vi "SGUI Search Control Ref.vi"(6 "error in":errorcluster, 8 "control label (empty)":string, 9 "generate error if not found? (True)":bool=TRUE) -> (7 "error out":errorcluster, 10 "found?":bool, 11 "control ref out":refnum<vi>)   [LabVIEW 2013, in "varilib.lvlib"]
doc: "This VI searches control reference by its label in the previously regitered list (see 'SGUI Register Controls').\nIf multiple controls with the same name are found the priority has the last registered.\n\nError input is ignored however by default it will generate error if control is not found."
uses:
  varilib.lvlib
  SGUI Global Var.vi
  <vilib>/Utility/error.llb/Error Cluster From Error Code.vi
  <vilib>/ErrorRing/Error Ring.xnode
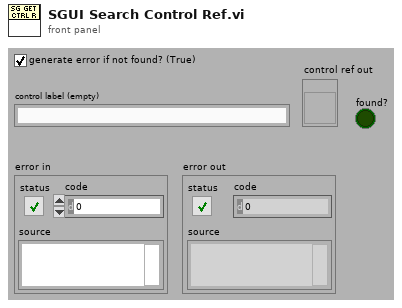
[diagram p1: front panel]
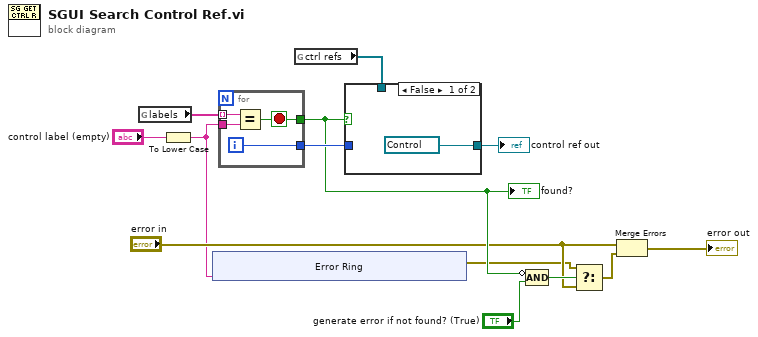
[diagram p0: block diagram]
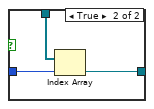
[diagram p2: hidden frame]
diagram:
  n1 = global read "SGUI Global Var.vi" "labels"() -> (w13:string[])
  n2 = To Lower Case(string="control label (empty)") -> (all lower case string=w1:string)
  n3 = xnode "Error Ring"("parameter 0"=w1) -> ("error out"=w2:errorcluster)
  n4 = for {
    tunnel: w13 -> [w17] mode=indexing
    tunnel: w1 -> [w16]
    tunnel: [w15] -> w11
    tunnel: [w14] -> w5
    i -> [w15]
    stop <- w14 stop-if-true
    n5 = Equal?(x=w17, y=w16) -> (x = y?=w14:bool)
  }
  "found?" <- w5
  n6 = global read "SGUI Global Var.vi" "ctrl refs"() -> (w12:refnum<vi>[])
  n7 = case shown="False" w5 {
    tunnel: w12 -> [_ w21]
    tunnel: w11 -> [_ w20]
    tunnel: [refnum<vi> refnum ("ctrl ref out") w19] -> w10
    frame False {
    }
    frame True {
      n8 = Index Array(array=w21, index=w20) -> (element=w19:refnum<vi>)
    }
  }
  "control ref out" <- w10
  n9 = Compound Arithmetic op=AND(invert w5, "generate error if not found? (True)") -> (w6:bool)
  n10 = Select(t=w2, s=w6, f="error in") -> (s? t:f=w7:errorcluster)
  n11 = Merge Errors("error in", w7) -> (→"error out":errorcluster)
